vi "CCWorklistSCUFilter.vi"(8 "error in (no error)":errorcluster, 10 "TimeCluster":T1, 11 ".NET Refnum in":refnum<k24>) -> (0 "error out":errorcluster)   [LabVIEW 2013, in "main.lvlib" / "ClearCanvasLibrary.lvlib"]
uses:
  ClearCanvasLibrary.lvlib
  C:/Users/Simon/SkyDrive/LabView/2013/DM2020/DICOM/ClearCanvasNewBuild/ClearCanvas.Dicom.dll
  ClearCanvasNewBuild/ClearCanvas.Dicom.dll
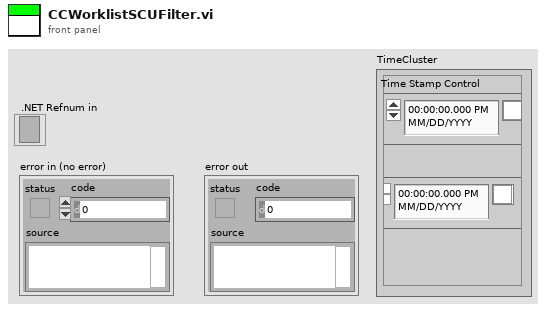
[diagram p1: front panel]
types:
  T1 = cluster{"Time Stamp Control":timestamp, "Time Stamp Control 2":timestamp}
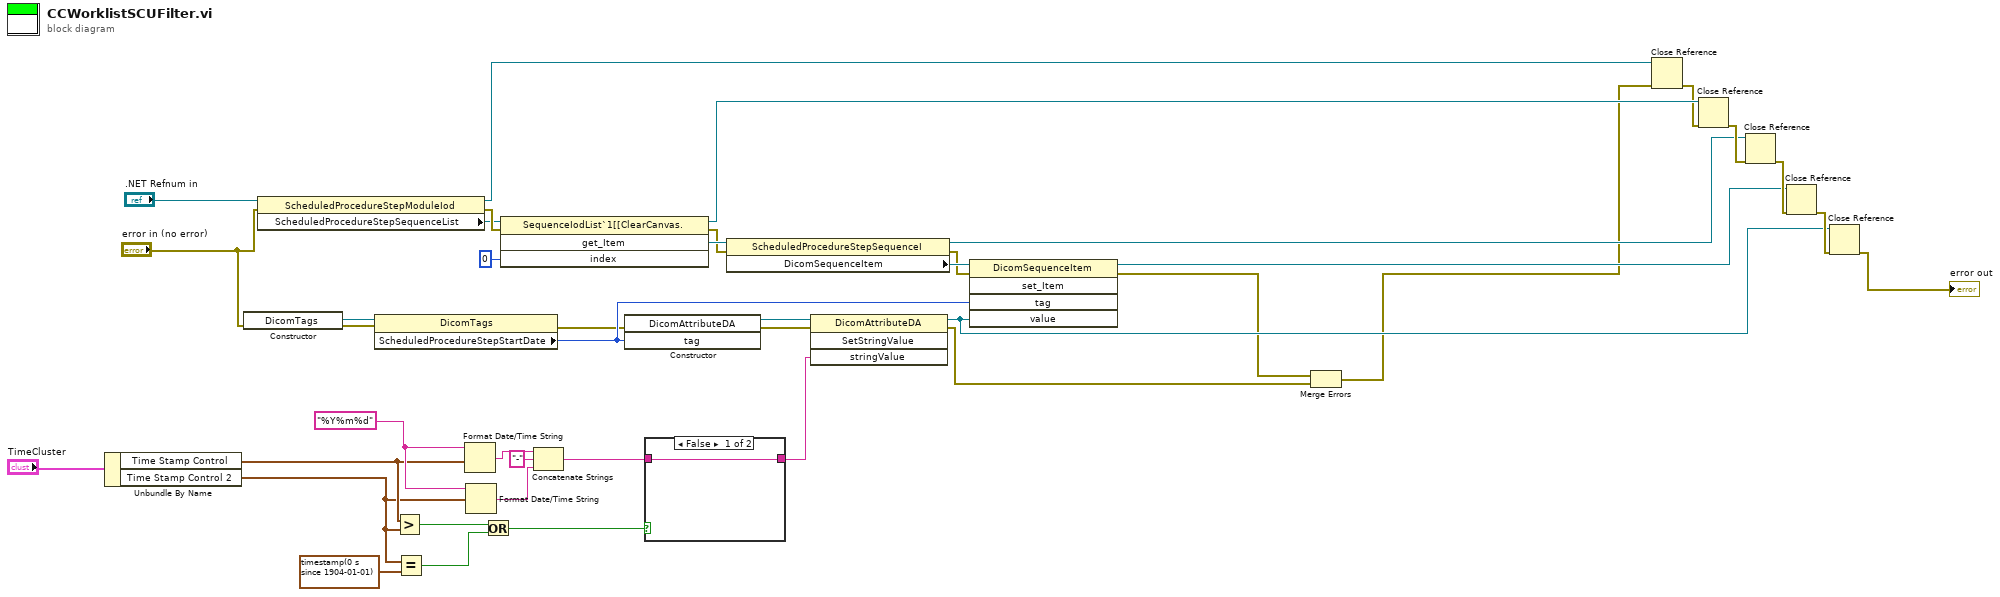
[diagram p0: block diagram]
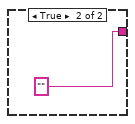
[diagram p2: hidden frame]
diagram:
  w18 = "%Y%m%d"
  n1 = Unbundle By Name("TimeCluster") -> ("Time Stamp Control"=w12:timestamp, "Time Stamp Control 2"=w10:timestamp)
  n2 = constructor class="DicomTags"(error in="error in (no error)") -> (reference out=w6:refnum<k24>, error out=w25:errorcluster)  [unwired: 2 in, 1 out]
  n3 = property class="ScheduledProcedureStepModuleIod"(reference=".NET Refnum in", error in="error in (no error)") -> (reference out=w37:refnum<k24>, error out=w41:errorcluster, "ScheduledProcedureStepSequenceList"=w40:refnum<k24>)
  n4 = property class="DicomTags"(reference=w6, error in=w25) -> (error out=w23:errorcluster, "ScheduledProcedureStepStartDate"=w30:u32)  [unwired: 1 out]
  n5 = Greater?(x=w12, y=w10) -> (0:w9:bool)
  n6 = Equal?(x=w10, y=timestamp(0 s since 1904-01-01)) -> (x = y?=w8:bool)
  n7 = Format Date/Time String(time format string (%c)=w18, seconds (now)=w12) -> (date/time string=w17:string)  [unwired: 1 in]
  n8 = Format Date/Time String(time format string (%c)=w18, seconds (now)=w10) -> (date/time string=w15:string)  [unwired: 1 in]
  n9 = Or(x=w9, y=w8) -> (x .or. y?=w7:bool)
  n10 = invoke class="SequenceIodList`1[[ClearCanvas." method="get_Item"(reference=w40, error in=w41, "index"=0) -> (reference out=w36:refnum<k24>, error out=w21:errorcluster, "get_Item"=w32:refnum<k24>)  [unwired: 1 in, 1 out]
  n11 = Concatenate Strings(w17, "-" ("string"), w15) -> (w14:string)
  n12 = constructor class="DicomAttributeDA"(error in=w23, "tag"=w30) -> (reference out=w29:refnum<k24>, error out=w22:errorcluster)  [unwired: 2 in, 2 out]
  n13 = case shown="False" w7 {
    tunnel: w14 -> [w42 _]
    tunnel: [w42 ""] -> w13
    frame False {
    }
    frame True {
    }
  }
  n14 = property class="ScheduledProcedureStepSequenceI"(reference=w32, error in=w21) -> (reference out=w28:refnum<k24>, error out=w20:errorcluster, "DicomSequenceItem"=w31:refnum<k24>)
  n15 = invoke class="DicomAttributeDA" method="SetStringValue"(reference=w29, error in=w22, "stringValue"=w13) -> (reference out=w19:refnum<k24>, error out=w4:errorcluster)  [unwired: 1 in, 2 out]
  n16 = invoke class="DicomSequenceItem" method="set_Item"(reference=w31, error in=w20, "tag"=w30, "value"=w19) -> (reference out=w5:refnum<k24>, error out=w3:errorcluster)  [unwired: 1 in, 3 out]
  n17 = Merge Errors(w3, w4) -> (w2:errorcluster)
  n18 = Close Reference(reference=w37, error in (no error)=w2) -> (error out=w35:errorcluster)
  n19 = Close Reference(reference=w36, error in (no error)=w35) -> (error out=w34:errorcluster)
  n20 = Close Reference(reference=w28, error in (no error)=w34) -> (error out=w27:errorcluster)
  n21 = Close Reference(reference=w5, error in (no error)=w27) -> (error out=w26:errorcluster)
  n22 = Close Reference(reference=w19, error in (no error)=w26) -> (error out=→"error out":errorcluster)
